vi "Msg.vi"(7 "Actor in":refnum<class "Actor.lvclass">, 11 "Event Last Ack Msg in":refnum<class "Event Last Ack Msg.lvclass">) -> (5 "Actor out":refnum<class "Actor.lvclass">)   [LabVIEW 2021, in "Event Last Ack.lvlib" / "Event Last Ack Msg.lvclass"]
uses:
  Event Last Ack Msg.lvclass
  Actor/Actor.lvclass
  Event Last Ack/Event Last Ack.lvclass
  Event Last Ack Msg.lvclass/Event Last Ack Msg.ctl
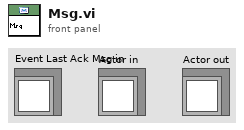
[diagram p1: front panel]
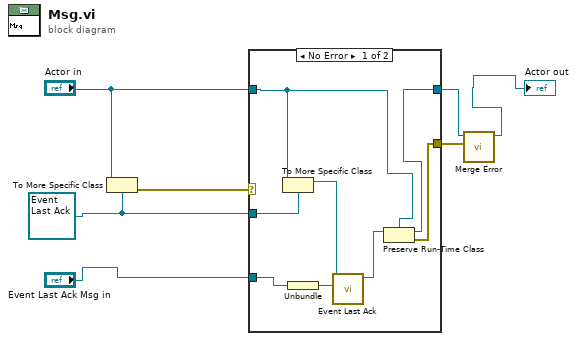
[diagram p0: block diagram]
diagram:
  w1 = refnum<class "Event Last Ack.lvclass"> refnum ("Event Last Ack.lvlib:Event Last Ack.lvclass")
  n1 = To More Specific Class(target class=w1, reference="Actor in") -> (error out=w7:errorcluster)  [unwired: 1 in, 1 out]
  n2 = case shown="No Error" w7 {
    selector: w7 -> [_ w16]
    tunnel: [w12 w17] -> w6
    tunnel: "Actor in" -> [w13 w17]
    tunnel: w1 -> [w15 _]
    tunnel: "Event Last Ack Msg in" -> [w14 _]
    tunnel: [w11 w16] -> w5
    frame No Error {
      n3 = To More Specific Class(target class=w15, reference=w13) -> (specific class reference=w9:refnum<class "Event Last Ack.lvclass">)  [unwired: 1 in, 1 out]
      n4 = Unbundle(w14) -> (w10:refnum<class "Event Actor.lvclass">)
      n5 = call-dynamic "Event Last Ack.vi"("Event Actor"=w10, "Event Last Ack in"=w9) -> ("Event Last Ack out"=w8:refnum<class "Event Last Ack.lvclass">)  [unwired: 9 in]
      n6 = Preserve Run-Time Class(object in=w8, 2:w13) -> (object out=w12:refnum<class "Actor.lvclass">, error out=w11:errorcluster)  [unwired: 1 in]
    }
    frame Error {
    }
  }
  n7 = call-dynamic "Merge Error.vi"("Error"=w5, "Set Error in"=w6) -> ("Set Error out"=→"Actor out":refnum<class "Actor.lvclass">)  [unwired: 9 in]
